vi "Configure.vi"(8 "error in":errorcluster, 9 "Config Handle":T1, 10 "section":string="Serial Config", 11 "Serial Session in":refnum<class "Serial Session.lvclass">) -> (0 "error out":errorcluster, 3 "Serial Session out":refnum<class "Serial Session.lvclass">)   [LabVIEW 2018, in "Serial Session.lvclass"]
doc: "Configure uses an existing configuration file association to configure the port for operation."
uses:
  Serial Session.lvclass
  C:/Program Files (x86)/National Instruments/LabVIEW 2018/user.lib/_Session Fwk/Session - Root.lvclass
  File Access/Config Data/Config Session.ctl
  File Access/Config Data/Config Data.lvclass
  Typedefs/Serial Config.ctl
  Typedefs/Msg Config.ctl
  Session Log/System Log.lvclass
  File Access/Config Data/Config Data.lvclass/Config Data.ctl
  Serial Session.lvclass/Serial Session.ctl
  Session Log/System Log.lvclass/System Log.ctl
  File Access/Config Data/Accessors/Read Ref.vi
  Session Log/Accessors/Write Main Path.vi
  Accessors/Write Sys Log.vi
  Accessors/Read Sys Log.vi
  Controller/xGlobal Data.vi
  <vilib>/Utility/config.llb/Read Key (I32).vi
  <vilib>/Utility/config.llb/Read Key (String).vi
  <userlib>/_Session Fwk/Accessors/_get Session Name for PN.vi
  <userlib>/_Session Fwk/Session - Root.lvclass
  <vilib>/Utility/config.llb/NI_LVConfig.lvlib
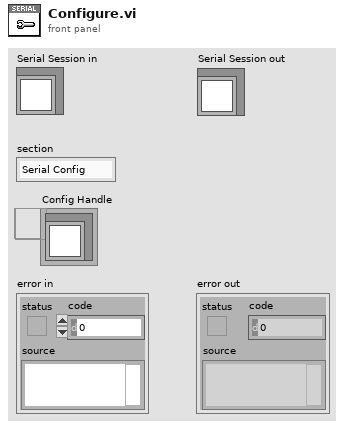
[diagram p1: front panel]
types:
  T1 = typedef "Config Data.lvclass/Config Session.ctl" = refnum<data-value>
  T2 = typedef "Serial Session.lvclass/Msg Config.ctl" = cluster{"sendEndEn":bool, "suppEnEnRd":bool, "termChar":u8, "EnTermChar":bool}
  T3 = typedef "Serial Session.lvclass/Serial Config.ctl" = cluster{"baud rate":u32, "data bits":u16, "stop bits":u16, "parity":u16, "flow control":u16, "endModeforReads":u16, "endModeforWrites":u16}
  T4 = typedef "NI_LVConfig.lvlib/Config Data RefNum.ctl" = refnum<k1>
  T5 = typedef "Session - Root.lvclass/Session Handle.ctl" = refnum<data-value>
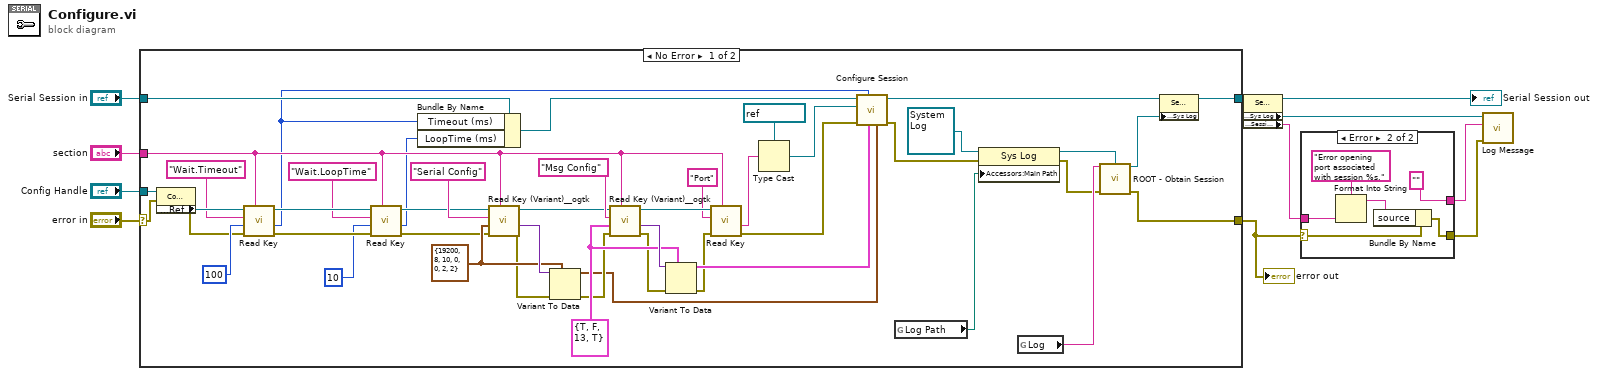
[diagram p0: block diagram]
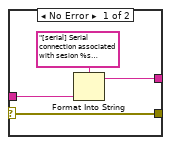
[diagram p2: hidden frame]
diagram:
  n1 = case shown="No Error" "error in" {
    selector: "error in" -> [w46 w59]
    tunnel: [w15 w59] -> w1
    tunnel: [w13 w58] -> w2
    tunnel: "Serial Session in" -> [w25 w58]
    tunnel: "Config Handle" -> [w57 _]
    tunnel: "section" -> [w32 _]
    frame No Error {
      w50 = T2 {"sendEndEn"=TRUE, "suppEnEnRd"=FALSE, "termChar"=13, "EnTermChar"=TRUE} ("Msg Configuration")
      w55 = T3 {"baud rate"=19200, "data bits"=8, "stop bits"=10, "parity"=0, "flow control"=0, "endModeforReads"=2, "endModeforWrites"=2} ("Serial Config")
      n2 = property class="Config Data"(reference=w57, error in=w46) -> (error out=w26:errorcluster, "Accessors:Ref"=w36:T4)  [unwired: 1 out]
      n3 = call-poly <vilib>:"Read Key.vi"("section"=w32, "error in (no error)"=w26, "default value"=100, "key"="Wait.Timeout", "refnum"=w36) -> ("error out"=w30:errorcluster, "value"=w22:i32, "refnum out"=w34:T4)  [unwired: 3 in, 1 out]
      n4 = call-poly <vilib>:"Read Key.vi"("section"=w32, "error in (no error)"=w30, "default value"=10, "key"="Wait.LoopTime", "refnum"=w34) -> ("error out"=w27:errorcluster, "value"=w23:i32, "refnum out"=w33:T4)  [unwired: 3 in, 1 out]
      n5 = Bundle By Name(cluster=w25, "Timeout (ms)"=w22, "LoopTime (ms)"=w23) -> (w24:refnum<class "Serial Session.lvclass">)
      n6 = call <userlib>:"Read Key (Variant)__ogtk.vi"("section"=w32, "error in (no error)"=w27, "type"=w55, "key (optional)"="Serial Config", "refnum"=w33) -> ("error out"=w54:errorcluster, "key-value"=w56:variant, "refnum out"=w45:T4)  [unwired: 3 in, 1 out]
      n7 = Variant To Data(error in=w54, type=w55, Variant=w56) -> (data=w40:T3, error out=w49:errorcluster)
      n8 = call <userlib>:"Read Key (Variant)__ogtk.vi"("section"=w32, "error in (no error)"=w49, "type"=w50, "key (optional)"="Msg Config", "refnum"=w45) -> ("error out"=w38:errorcluster, "key-value"=w51:variant, "refnum out"=w48:T4)  [unwired: 3 in, 1 out]
      n9 = Variant To Data(error in=w38, type=w50, Variant=w51) -> (data=w39:T2, error out=w37:errorcluster)
      n10 = call-poly <vilib>:"Read Key.vi"("section"=w32, "error in (no error)"=w37, "key"="Port", "refnum"=w48) -> ("error out"=w42:errorcluster, "value"=w44:string)  [unwired: 4 in, 2 out]
      n11 = Type Cast(type=refnum<visa-resource-name> "COM5" ("VISA Resource"), x=w44) -> (*(type *) &x=w41:refnum<visa-resource-name>)
      n12 = call "Configure Session.vi"("serialCfg"=w40, "Message Cfg"=w39, "timeout"=w22, "error in"=w42, "VISA Resource"=w41, "Serial Session"=w24) -> ("error out"=w17:errorcluster, "Serial Session out"=w14:refnum<class "Serial Session.lvclass">)  [unwired: 4 in]
      n13 = global read "xGlobal Data.vi" "Log Path"() -> (w20:path)
      n14 = property class="Sys Log"(reference=refnum<class "System Log.lvclass"> refnum ("Sys Log"), error in=w17, "Accessors:Main Path"=w20) -> (reference out=w19:refnum<class "System Log.lvclass">, error out=w16:errorcluster)
      n15 = global read "xGlobal Data.vi" "Log"() -> (w18:string)
      n16 = call <userlib>:"ROOT - Obtain Session.vi"("Session Name ()"=w18, "OBJ - Session"=w19, "error in (no error)"=w16) -> ("Session Handle"=w12:T5, "error out"=w15:errorcluster)  [unwired: 10 in, 1 out]
      n17 = property class="Serial Session"(reference=w14, "Public:Accessors:Sys Log"=w12) -> (reference out=w13:refnum<class "Serial Session.lvclass">)  [unwired: 1 in, 1 out]
    }
    frame Error {
    }
  }
  "error out" <- w1
  n18 = property class="Serial Session"(reference=w2) -> (reference out=→"Serial Session out":refnum<class "Serial Session.lvclass">, "Public:Accessors:Sys Log"=w5:T5, "Accessors:Session Name"=w7:string)  [unwired: 1 in, 1 out]
  n19 = case shown="Error" w1 {
    selector: w1 -> [w60 w69]
    tunnel: w7 -> [w62 w67]
    tunnel: [w61 ""] -> w6
    tunnel: [w60 w65] -> w4
    frame No Error {
      n20 = Format Into String(format string="[serial] Serial connection associated with sesion %s opened.", w62) -> (resulting string=w61:string)  [unwired: 2 in, 1 out]
    }
    frame Error {
      n21 = Format Into String(format string="Error opening port associated with session %s." ("source"), w67) -> (resulting string=w66:string)  [unwired: 2 in, 1 out]
      n22 = Bundle By Name(cluster=w69, "source"=w66) -> (w65:errorcluster)
    }
  }
  n23 = call "Log Message.vi"("error in"=w4, "MSG In"=w6, "session in"=w5) -> ()  [unwired: 7 in, 2 out]
